vi "Make ramp data.vi"(5 "gap time (s)":dbl, 6 "randomize":bool=TRUE, 7 "Repetitions":i32=2, 8 "Hold time (s)":dbl[](array[numeric]), 9 "Directions":dbl[](array[numeric])=[1.0, -1.0], 10 "Ramp velocities (deg/s)":dbl[](array[numeric])=[5.0, 10.0], 11 "Final positions (deg)":dbl[](array[numeric])=[5.0, 10.0, 20.0]) -> (2 "Total time":dbl, 3 "ramp data":T1)   [LabVIEW 2013]
uses:
  Pulse data.ctl
  <vilib>/gmath/statdist.llb/Random Permutation.vi
  <vilib>/gmath/NI_Gmath.lvlib
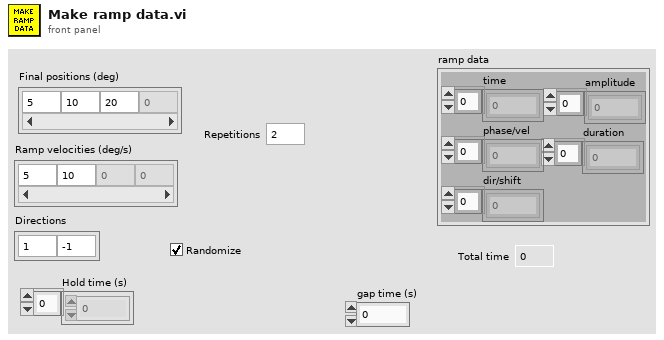
[diagram p1: front panel]
types:
  T1 = typedef "Pulse data.ctl" = cluster{"time":dbl[], "phase/vel":dbl[], "dir/shift":dbl[], "amplitude":dbl[], "duration":dbl[]}
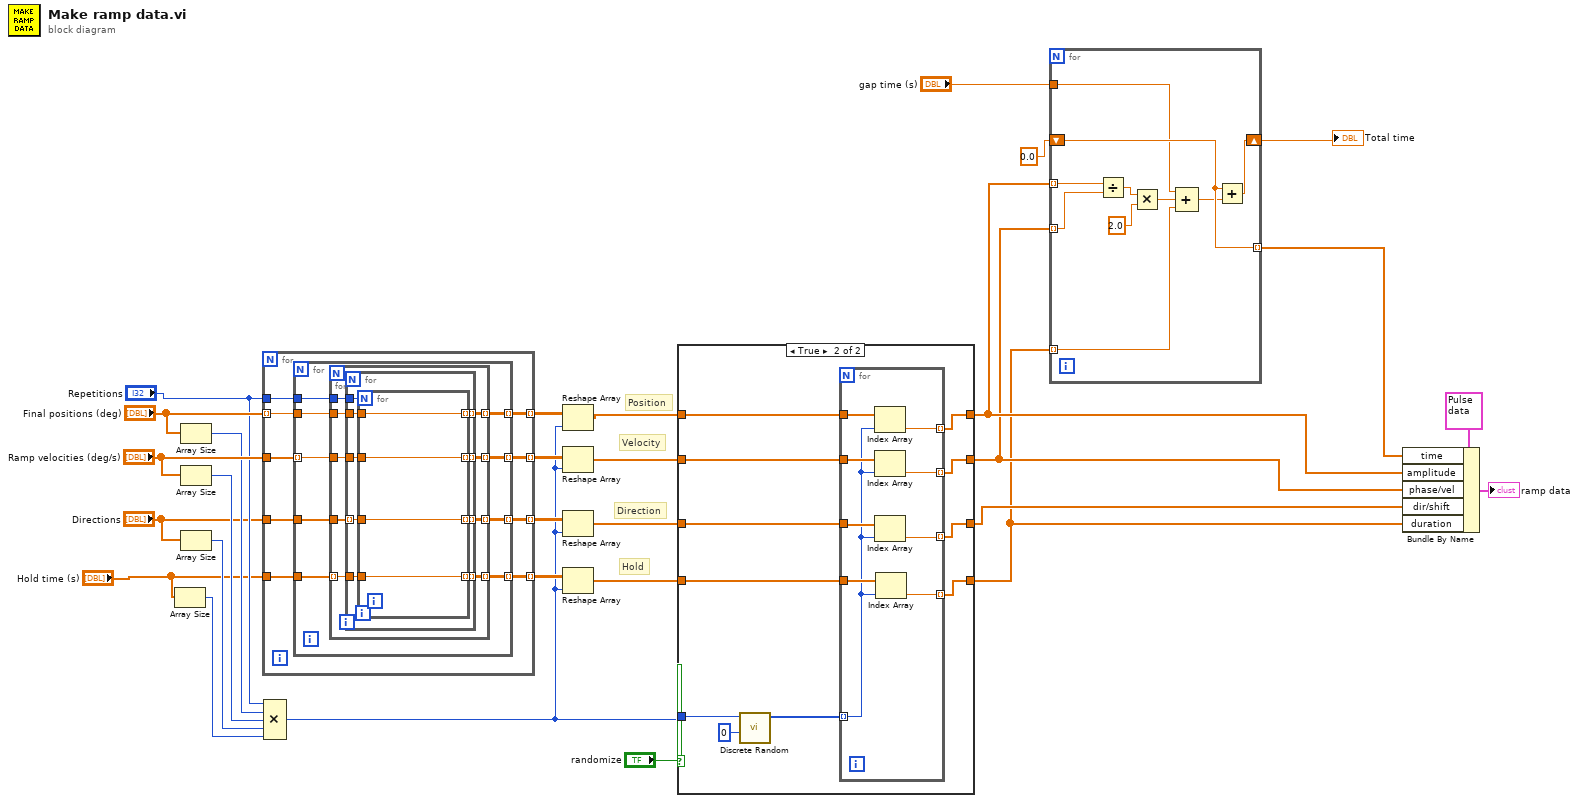
[diagram p0: block diagram]
diagram:
  # "Hold"
  # "Direction"
  # "Velocity"
  # "Position"
  n1 = Array Size(array="Hold time (s)") -> (size(s)=w20:i32)
  n2 = Array Size(array="Final positions (deg)") -> (size(s)=w26:i32)
  n3 = Array Size(array="Ramp velocities (deg/s)") -> (size(s)=w25:i32)
  n4 = Array Size(array="Directions") -> (size(s)=w19:i32)
  n5 = for {
    tunnel: "Final positions (deg)" -> [w36] mode=indexing
    tunnel: "Ramp velocities (deg/s)" -> [w38]
    tunnel: "Hold time (s)" -> [w37]
    tunnel: [w35] -> w23 mode=indexing
    tunnel: [w34] -> w24 mode=indexing
    tunnel: [w33] -> w22 mode=indexing
    tunnel: "Repetitions" -> [w32]
    tunnel: "Directions" -> [w31]
    tunnel: [w30] -> w18 mode=indexing
    n6 = for {
      tunnel: w38 -> [w45] mode=indexing
      tunnel: w37 -> [w47]
      tunnel: w36 -> [w46]
      tunnel: [w44] -> w35 mode=indexing
      tunnel: [w43] -> w34 mode=indexing
      tunnel: [w42] -> w33 mode=indexing
      tunnel: w32 -> [w41]
      tunnel: w31 -> [w40]
      tunnel: [w39] -> w30 mode=indexing
      n7 = for {
        tunnel: w47 -> [w54] mode=indexing
        tunnel: w46 -> [w56]
        tunnel: w45 -> [w55]
        tunnel: [w52] -> w43 mode=indexing
        tunnel: [w51] -> w44 mode=indexing
        tunnel: [w50] -> w42 mode=indexing
        tunnel: w41 -> [w53]
        tunnel: w40 -> [w49]
        tunnel: [w48] -> w39 mode=indexing
        n8 = for {
          tunnel: w56 -> [w65]
          tunnel: w55 -> [w64]
          tunnel: w54 -> [w63]
          tunnel: w53 -> [w62]
          tunnel: [w61] -> w52 mode=indexing
          tunnel: [w60] -> w51 mode=indexing
          tunnel: [w59] -> w50 mode=indexing
          tunnel: w49 -> [w58] mode=indexing
          tunnel: [w57] -> w48 mode=indexing
          n9 = for {
            N: w62 -> [_]
            tunnel: w65 -> [w69]
            tunnel: w64 -> [w68]
            tunnel: w63 -> [w67]
            tunnel: [w69] -> w61 mode=indexing
            tunnel: [w68] -> w60 mode=indexing
            tunnel: [w67] -> w59 mode=indexing
            tunnel: w58 -> [w66]
            tunnel: [w66] -> w57 mode=indexing
          }
        }
      }
    }
  }
  n10 = Compound Arithmetic op=MULTIPLY("Repetitions", w26, w25, w19, w20) -> (w4:i32)
  n11 = Reshape Array(w24, w4) -> (w16:dbl[])
  n12 = Reshape Array(w23, w4) -> (w15:dbl[])
  n13 = Reshape Array(w18, w4) -> (w14:dbl[])
  n14 = Reshape Array(w22, w4) -> (w13:dbl[])
  n15 = case shown="True" "randomize" {
    tunnel: w4 -> [_ w83]
    tunnel: w16 -> [w73 w82]
    tunnel: w15 -> [w72 w81]
    tunnel: [w73 w78] -> w9
    tunnel: [w72 w79] -> w8
    tunnel: w14 -> [w71 w77]
    tunnel: w13 -> [w70 w76]
    tunnel: [w71 w75] -> w7
    tunnel: [w70 w74] -> w6
    frame False {
    }
    frame True {
      n16 = call-poly <vilib>:"Discrete Random.vi"("start"=0, "N"=w83) -> ("random permutation"=w80:i32[])  [unwired: 8 in, 1 out]
      n17 = for {
        tunnel: w82 -> [w93]
        tunnel: w81 -> [w92]
        tunnel: w80 -> [w87] mode=indexing
        tunnel: [w91] -> w78 mode=indexing
        tunnel: [w90] -> w79 mode=indexing
        tunnel: w77 -> [w88]
        tunnel: w76 -> [w89]
        tunnel: [w86] -> w75 mode=indexing
        tunnel: [w85] -> w74 mode=indexing
        n18 = Index Array(array=w93, index=w87) -> (element=w91:dbl)
        n19 = Index Array(array=w92, index=w87) -> (element=w90:dbl)
        n20 = Index Array(array=w88, index=w87) -> (element=w86:dbl)
        n21 = Index Array(array=w89, index=w87) -> (element=w85:dbl)
      }
    }
  }
  n22 = for {
    tunnel: w9 -> [w103] mode=indexing
    tunnel: w8 -> [w102] mode=indexing
    tunnel: w6 -> [w95] mode=indexing
    shift-right: [w99] -> w1
    shift-left: 0.0 -> [w98]
    tunnel: [w98] -> w10 mode=indexing
    tunnel: "gap time (s)" -> [w94]
    n23 = Divide(x=w103, y=w102) -> (x/y=w97:dbl)
    n24 = Multiply(x=w97, y=2.0) -> (x*y=w100:dbl)
    n25 = Compound Arithmetic op=ADD(w94, w100, w95) -> (w96:dbl)
    n26 = Add(x=w98, y=w96) -> (x+y=w99:dbl)
  }
  "Total time" <- w1
  n27 = Bundle By Name(cluster=T1 {"time"=[0.2222222222222222, 6.888888888888888, 13.333333333333332, 20.22222222222222, 26.666666666666664, 33.77777777777777, 40.44444444444444, 46.666666666666664, 53.77777777777777, 59.99999999999999, 66.88888888888889, 73.77777777777777], "phase/vel"=[0.3333333333333333, 0.3333333333333333, 0.0, 0.3333333333333333, 0.0, 0.6666666666666666, 0.6666666666666666, 0.0, 0.6666666666666666, 0.0, 0.3333333333333333, 0.6666666666666666], "dir/shift"=[1.0, -1.0, -1.0, 1.0, 1.0, -1.0, -1.0, -1.0, 1.0, 1.0, -1.0, 1.0], "amplitude"=[5.0, 5.0, 5.0, 5.0, 5.0, 5.0, 5.0, 5.0, 5.0, 5.0, 5.0, 5.0], "duration"=[0.2, 0.2, 0.2, 0.2, 0.2, 0.2, 0.2, 0.2, 0.2, 0.2, 0.2, 0.2]} ("pulse data 2"), "time"=w10, "amplitude"=w9, "phase/vel"=w8, "dir/shift"=w7, "duration"=w6) -> (→"ramp data":T1)
